vi "LabviewIngestService CreateIngestionConfig.vi"(6 "contextId":T1, 8 "error in":errorcluster, 9 "timeout (ms)":i32=-1, 10 "Request Data":T3, 11 "gRPC ID":T1) -> (0 "error out":errorcluster, 2 "Response Data":T2, 3 "gRPC ID out":T1)   [LabVIEW 2024, in "SiftProxy_client.lvlib"]
uses:
  SiftProxy_client.lvlib
  <vilib>/gRPC/LabVIEW gRPC Library/Shared/grpcId.ctl
  RPC Messages/sift_proxy_v1_CreateLabviewIngestionConfigRequest.ctl
  RPC Messages/sift_proxy_v1_ChannelConfig.ctl
  RPC Messages/sift_proxy_v1_ChannelDataType.ctl
  RPC Messages/sift_proxy_v1_ChannelEnumType.ctl
  RPC Messages/sift_proxy_v1_ChannelBitFieldElement.ctl
  RPC Messages/sift_proxy_v1_CreateLabviewIngestionConfigResponse.ctl
  RPC Messages/sift_proxy_v1_CreateLabviewIngestionConfigResponse_Flat.ctl
  14035477-4c25-4107-8ed5-d0c4ef420ce5.vi
  RPC Messages/RichToFlatsift_proxy_v1_ChannelConfig.vi
  <vilib>/gRPC/LabVIEW gRPC Library/Shared/TranslateGrpcError.vi
  <vilib>/gRPC/LabVIEW gRPC Library/Shared/Wait On Occurrence Wrapper.vi
  RPC Messages/RichToFlatsift_proxy_v1_ChannelEnumType.vi
  RPC Messages/RichToFlatsift_proxy_v1_ChannelBitFieldElement.vi
  <vilib>/gRPC/LabVIEW gRPC Library/Shared/Wait On Occurence.vi
  <vilib>/gRPC/LabVIEW gRPC Library/Server API/Server/Get Server DLL Path.vi
  <vilib>/Utility/error.llb/Error Cluster From Error Code.vi
  <vilib>/Utility/config.llb/Open Config Data.vi
  <vilib>/Utility/config.llb/Write Key.vi
  <vilib>/Utility/config.llb/Write Key (Boolean).vi
  <vilib>/Utility/config.llb/Not A Config Data Refnum.vi
  <vilib>/Utility/config.llb/Read Key.vi
  <vilib>/Utility/config.llb/Read Key (Boolean).vi
  <vilib>/Utility/config.llb/Close Config Data.vi
  <vilib>/gRPC/LabVIEW gRPC Library/grpc-lvsupport-release.lvlib
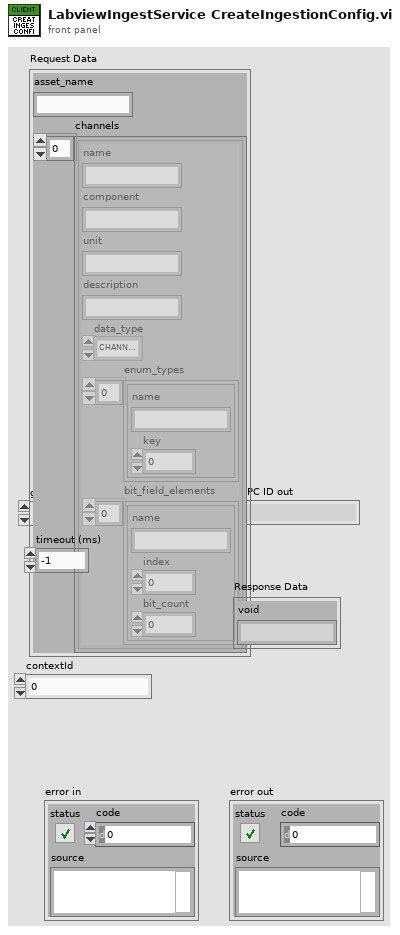
[diagram p1: front panel]
types:
  T1 = typedef "grpc-lvsupport-release.lvlib/grpcId.ctl" = u64
  T2 = typedef "SiftProxy_client.lvlib/sift_proxy_v1_CreateLabviewIngestionConfigResponse.ctl" = cluster{"void":string}
  T3 = typedef "SiftProxy_client.lvlib/sift_proxy_v1_CreateLabviewIngestionConfigRequest.ctl" = cluster{"asset_name":string, "channels":T4[]}
  T4 = typedef "SiftProxy_client.lvlib/sift_proxy_v1_ChannelConfig.ctl" = cluster{"name":string, "component":string, "unit":string, "description":string, "data_type":T5, "enum_types":T6[], "bit_field_elements":T7[]}
  T5 = typedef "SiftProxy_client.lvlib/sift_proxy_v1_ChannelDataType.ctl" = enum32{"CHANNEL_DATA_TYPE_UNSPECIFIED", "CHANNEL_DATA_TYPE_DOUBLE", "CHANNEL_DATA_TYPE_STRING", "CHANNEL_DATA_TYPE_ENUM", "CHANNEL_DATA_TYPE_BIT_FIELD", "CHANNEL_DATA_TYPE_BOOL", "CHANNEL_DATA_TYPE_FLOAT", "CHANNEL_DATA_TYPE_INT_32", "CHANNEL_DATA_TYPE_UINT_32", "CHANNEL_DATA_TYPE_INT_64", "CHANNEL_DATA_TYPE_UINT_64"}
  T6 = typedef "SiftProxy_client.lvlib/sift_proxy_v1_ChannelEnumType.ctl" = cluster{"name":string, "key":u32}
  T7 = typedef "SiftProxy_client.lvlib/sift_proxy_v1_ChannelBitFieldElement.ctl" = cluster{"name":string, "index":i32, "bit_count":u32}
  T8 = typedef "SiftProxy_client.lvlib/sift_proxy_v1_CreateLabviewIngestionConfigResponse_Flat.ctl" = cluster{"void":string}
  T9 = typedef "SiftProxy_client.lvlib/sift_proxy_v1_CreateLabviewIngestionConfigRequest_Flat.ctl" = cluster{"asset_name":string, "channels":T10[]}
  T10 = typedef "SiftProxy_client.lvlib/sift_proxy_v1_ChannelConfig_Flat.ctl" = cluster{"name":string, "component":string, "unit":string, "description":string, "data_type":T5, "enum_types":T11[], "bit_field_elements":T12[]}
  T11 = typedef "SiftProxy_client.lvlib/sift_proxy_v1_ChannelEnumType_Flat.ctl" = cluster{"name":string, "key":u32}
  T12 = typedef "SiftProxy_client.lvlib/sift_proxy_v1_ChannelBitFieldElement_Flat.ctl" = cluster{"name":string, "index":i32, "bit_count":u32}
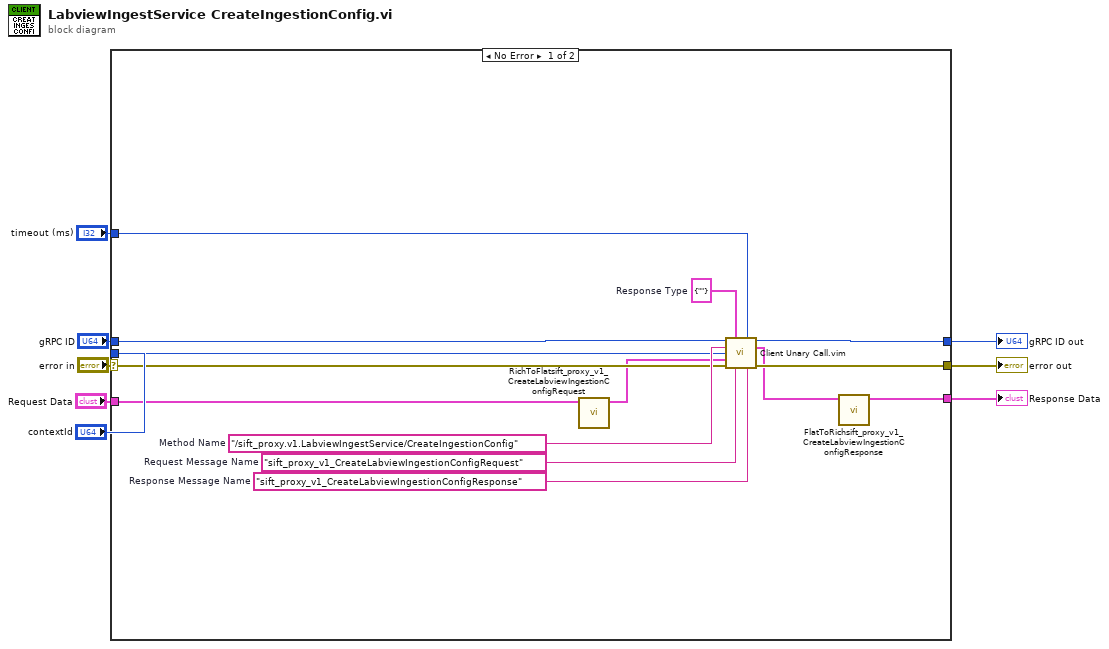
[diagram p0: block diagram]
diagram:
  n1 = case shown="No Error" "error in" {
    selector: "error in" -> [w18 w23]
    tunnel: [w17 w23] -> w7
    tunnel: "gRPC ID" -> [w16 w24]
    tunnel: [w15 w24] -> w5
    tunnel: "Request Data" -> [w12 _]
    tunnel: [w9 _] -> w3
    tunnel: "timeout (ms)" -> [w14 _]
    tunnel: "contextId" -> [w13 _]
    frame No Error {
      w19 = "sift_proxy_v1_CreateLabviewIngestionConfigResponse"  # Response Message Name
      w20 = "sift_proxy_v1_CreateLabviewIngestionConfigRequest"  # Request Message Name
      w21 = T8 {"void"=""}  # Response Type
      w22 = "/sift_proxy.v1.LabviewIngestService/CreateIngestionConfig"  # Method Name
      n2 = call "RichToFlatsift_proxy_v1_CreateLabviewIngestionConfigRequest.vi"("InputCluster"=w12) -> ("OutputCluster"=w11:T9)  [unwired: 10 in]
      n3 = call "Client Unary Call.vim"("ClientID in"=w16, "Response Type"=w21, "timeout (ms)"=w14, "Method Name"=w22, "contextId"=w13, "Request Data"=w11, "error in"=w18, "Request Message Name"=w20, "Response Message Name"=w19) -> ("ClientID out"=w15:u64, "Response Data"=w10:T8, "error out"=w17:errorcluster)  [unwired: 4 in]
      n4 = call "FlatToRichsift_proxy_v1_CreateLabviewIngestionConfigResponse.vi"("InputCluster"=w10) -> ("OutputCluster"=w9:T2)  [unwired: 10 in]
    }
    frame Error {
    }
  }
  "error out" <- w7
  "gRPC ID out" <- w5
  "Response Data" <- w3
